vi "DigitalConversion.vi"(0 "Amplitude(V)":dbl=1.0 format="%#_13g") -> (4 "Rise time":dbl format="%#_6p", 6 "Fall time":dbl format="%#_6p", 8 "High Peak":dbl, 10 "Low Peak":dbl, 13 "Input Analog Signal":waveform(dbl)(graph)={"t0"=timestamp(0 s since 1904-01-01), "dt"=1e-06, "Y"=array[10000 elements]}, 15 "Comparison":cluster{dbl, i16}(graph))   [LabVIEW 2020]
doc: "This VI is used to convert a pulsating square wave into a perfect digital signal and measures the maximum minimum and the rise time and fall time of the signal"
panel:
  out "Output Digital Waveform":digitaldata(graph)
  # "Analog to Digital Conversion"
  # "This Vi gets the distored square waveform and converts it to digital output in three different range:\nLess than 30%\nGreater than 70%\nBetween 30 and 70%"
  # "INPUT"
  # "OUTPUT"
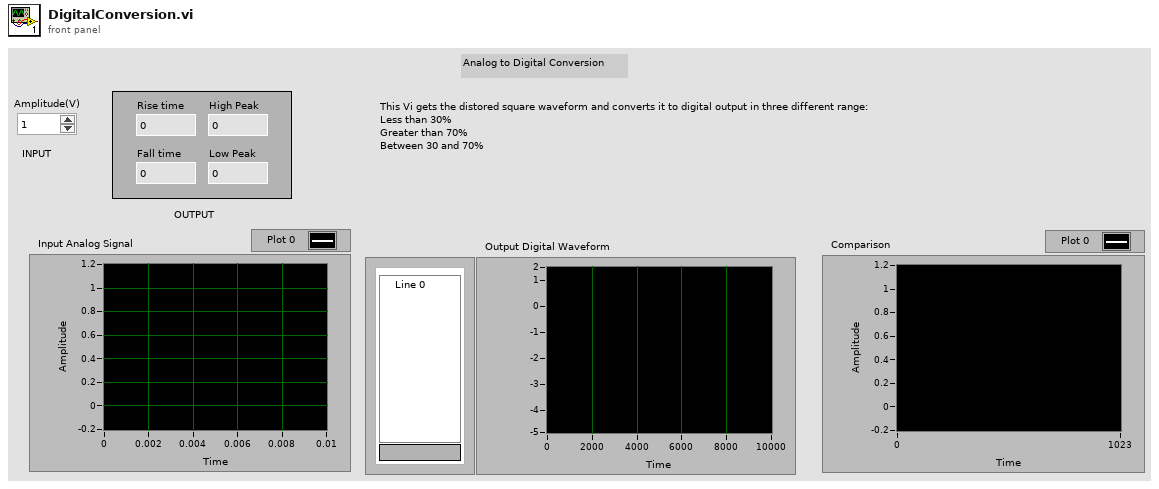
[diagram p1: front panel]
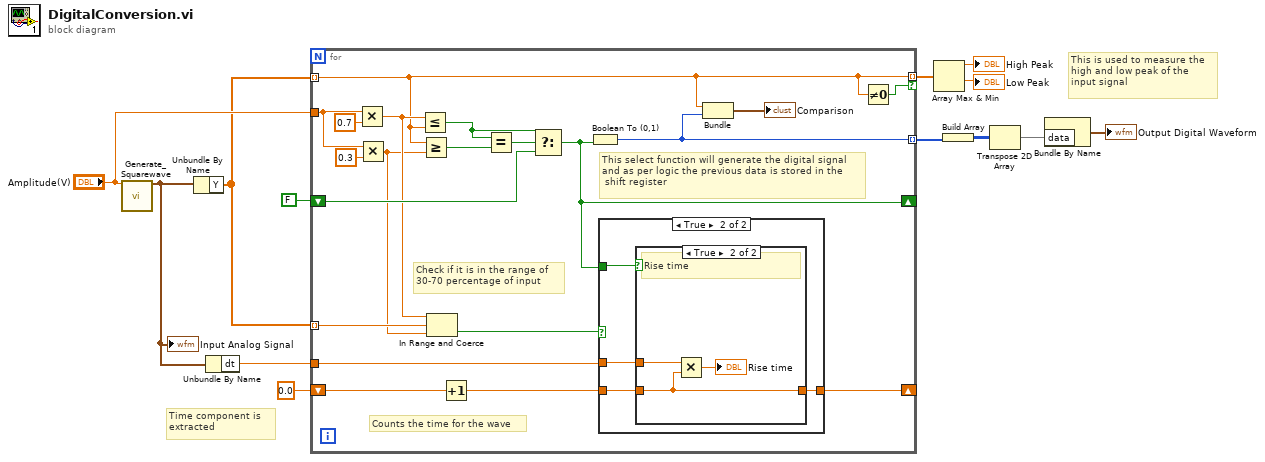
[diagram p0: block diagram]
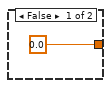
[diagram p2: hidden frame]
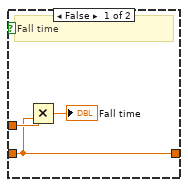
[diagram p3: hidden frame]
diagram:
  # "Time component is \nextracted"
  # "This is used to measure the \nhigh and low peak of the \ninput signal"
  n1 = call "Generate_Squarewave.vi"("Amplitude(V)"="Amplitude(V)") -> ("Waveform_Out"=w5:waveform(dbl))  [unwired: 13 in, 1 out]
  "Input Analog Signal" <- w5
  n2 = Unbundle By Name(w5) -> ("Y"=w11:dbl[])
  n3 = Unbundle By Name(w5) -> ("dt"=w10:dbl)
  n4 = for {
    tunnel: "Amplitude(V)" -> [w32]
    shift-right: [w17] -> _
    shift-left: FALSE -> [w29]
    tunnel: w11 -> [w16] mode=indexing
    tunnel: w11 -> [w28] mode=indexing
    shift-right: [w25] -> _
    shift-left: 0.0 -> [w24]
    tunnel: w10 -> [w26]
    tunnel: [w16] -> w8 mode=indexing if=w18
    tunnel: [w14] -> w4 mode=indexing
    # "Counts the time for the wave"
    # "Check if it is in the range of \n30-70 percentage of input"
    # "This select function will generate the digital signal\nand as per logic the previous data is stored in the\n shift register"
    n5 = Multiply(x=w32, y=0.7) -> (x*y=w20:dbl)
    n6 = Multiply(x=w32, y=0.3) -> (x*y=w19:dbl)
    n7 = Less Or Equal?(x=w20, y=w16) -> (x <= y?=w21:bool)
    n8 = Greater Or Equal?(x=w16, y=w19) -> (x >= y?=w22:bool)
    n9 = In Range and Coerce(upper limit=w20, x=w28, lower limit=w19) -> (In Range?=w27:bool)  [unwired: 1 out]
    n10 = Increment(x=w24) -> (x+1=w23:dbl)
    n11 = Equal?(x=w21, y=w22) -> (x = y?=w30:bool)
    n12 = Select(t=w21, s=w30, f=w29) -> (s? t:f=w17:bool)
    n13 = Boolean To (0,1)(Boolean=w17) -> (0, 1=w14:i16)
    n14 = case shown="True" w27 {
      tunnel: w17 -> [_ w38]
      tunnel: w26 -> [_ w37]
      tunnel: [0.0 w35] -> w25
      tunnel: w23 -> [_ w36]
      frame False {
      }
      frame True {
        n15 = case shown="True" w38 {
          tunnel: w37 -> [w41 w44]
          tunnel: w36 -> [w39 w43]
          tunnel: [w39 w43] -> w35
          frame False {
            # "Fall time"
            n16 = Multiply(x=w41, y=w39) -> (x*y=→"Fall time":dbl)
          }
          frame True {
            # "Rise time"
            n17 = Multiply(x=w44, y=w43) -> (x*y=→"Rise time":dbl)
          }
        }
      }
    }
    n18 = Bundle(w16, w14) -> (→"Comparison":cluster{dbl, i16})  [unwired: 1 in]
    n19 = Not Equal To 0?(x=w16) -> (x != 0?=w18:bool)
  }
  n20 = Array Max & Min(array=w8) -> (max value=→"High Peak":dbl, min value=→"Low Peak":dbl)  [unwired: 2 out]
  n21 = Build Array(w4) -> (w3:i16[][])
  n22 = Transpose 2D Array(2D array=w3) -> (transposed array=w2:i16[][])
  n23 = Bundle By Name("data"=w2) -> (→"Output Digital Waveform":digitaldata)  [unwired: 1 in]
